vi "CW_change.vi"() -> ()   [LabVIEW 2020]
uses:
  SubVI/Fitting/fit.ctl
  SubVI/Microwave/mw.ctl
  SubVI/Fitting/fit_result.ctl
  <vilib>/Analysis/baseanly.llb/Mean (DBL).vi
  labview_control/Global  Parameter.vi
  labview_control/LaoJi/NI CTR/NI DAQ Counter.lvlib
  Labview Library/Libraries/ASG8100CY/ASG8100CY.lvlib
  <vilib>/Analysis/NI_AALBase.lvlib
panel:
  in  "milliseconds to wait":u32=20
  in  "等待时间（毫秒）":u32=200
  in  "Thre 2":dbl=82866.0 caption="counts" format="%0.2f"
  out "Fre step":ext
  out "Stop Ref":refnum<vi>
  out "x-y 2":dbl
  out "x-y":dbl
  out "error out":errorcluster
  in  "pulse loop times":i32=900000 format="%#.4p"
  out "Signal data":ext[](array[numeric])
  out "Pro data":ext[](array[numeric])
  out "Ref data":ext[](array[numeric])
  out "Fre sequence":ext[](array[numeric])=[1150.0, 1160.0, 1170.0, 1180.0, 1190.0, 1200.0, 1210.0, 1220.0, 1230.0, 1240.0, 1250.0, 1260.0, 1270.0, 1280.0, 1290.0, 1300.0, 1310.0, 1320.0, 1330.0, 1340.0, 1350.0, 1360.0, 1370.0, 1380.0, 1390.0, 1400.0, 1410.0, 1420.0, 1430.0, 1440.0, 1450.0, 1460.0, 1470.0, 1480.0, 1490.0, 1500.0, 1510.0, 1520.0, 1530.0, 1540.0, 1550.0, 1560.0, 1570.0, 1580.0, 1590.0, 1600.0, 1610.0, 1620.0, 1630.0, 1640.0]
  out "fit result":T1={"1/2pi"=0.0, "pi"=0.0, "3/2pi"=0.0, "T2"=0.0, "freq"=2869.360957411588, "gap"=0.0, "snr"=10.094902959180725, "width 2"=0.0, "freq 2"=0.0}
  out "element":dbl=2870.0
  in  "?":T2(tab)
  in  "CW Sequence Filepath":path=path "F:/Labview_Control_SIC/ASG8100_Labview/cw.pulse"
  in  "cw loop times":i32=1000 format="%#.4p"
  in  "Pulse Sequence Filepath":path
  out "freq":dbl
  out "freq 3":dbl=1434.680478705794
  out "Reference":cluster{"Fre sequence":ext[], "Ref data":ext[]}(graph)
  out "Signal":T3(graph) caption="signal"
  out "Sum of 3 Gaussians":T4(graph) caption="CW"
  out "Probability":cluster{"Fre sequence":ext[], "Pro data":ext[]}(graph) caption="CW"
  in  "?":T5=enum."cw_single_peak"
  in  "Limit":T6={"width threshold -"=2.0, "width threshold +"=8.0, "contrast threshold"=0.03, "fit error threshold"=3.0}
  out "NV or not?":bool
  in  "MW":T7={"mw_source"=enum."rigol", "MW Source IP Address"="192.168.3.3", "Remote Port"=5025, "Frequency(MHz)"=1500.0, "Power(dBm)"=-20.0}
  in  "setting section":T8={"mode"=enum."CW", "Start freq"=1150.0, "Stop freq"=1650.0, "Num Pts"=50, " dBm"=-15.0, "average"=3000, "Reference"=1}
  in  "Final Power dBm":dbl=-30.0
  out "fit frequency":dbl=2869.360957411588
  in  "freq offset":dbl
  in  "ratio":dbl=0.7
  out "Peak Count Rate":dbl=393329.896735343
  out "threshold":dbl=68289.2
  out "mean":dbl=82866.0 caption="counts" format="%0.2f"
  in  "autotrace\nbefore CW?":bool=TRUE
  in  "scan width":dbl=50.0
  in  "auto change":bool
  in  "drift(MHz)":ext
  in  "name":string="NV_1.17_"
  out "cw path":path=path "D:/cw data/NV_1.17_4_2_2021_5_06_50_PM.txt"
  in  "?":bool
  out "gap":dbl
  out "freq 2":dbl
  out "full name":string="NV_1.17_4_2_2021_5_06_50_PM"
  out "1-D Array of Real":dbl[](array[numeric])
  out "System Waveform Chart":u32[](graph)
  out "CW Chart":dbl(graph)
  out "Signal and Ref":cluster{"Numeric":dbl, "Numeric":dbl}(graph)
  # "auto change section"
  # "autotrace section"
  # "final section"
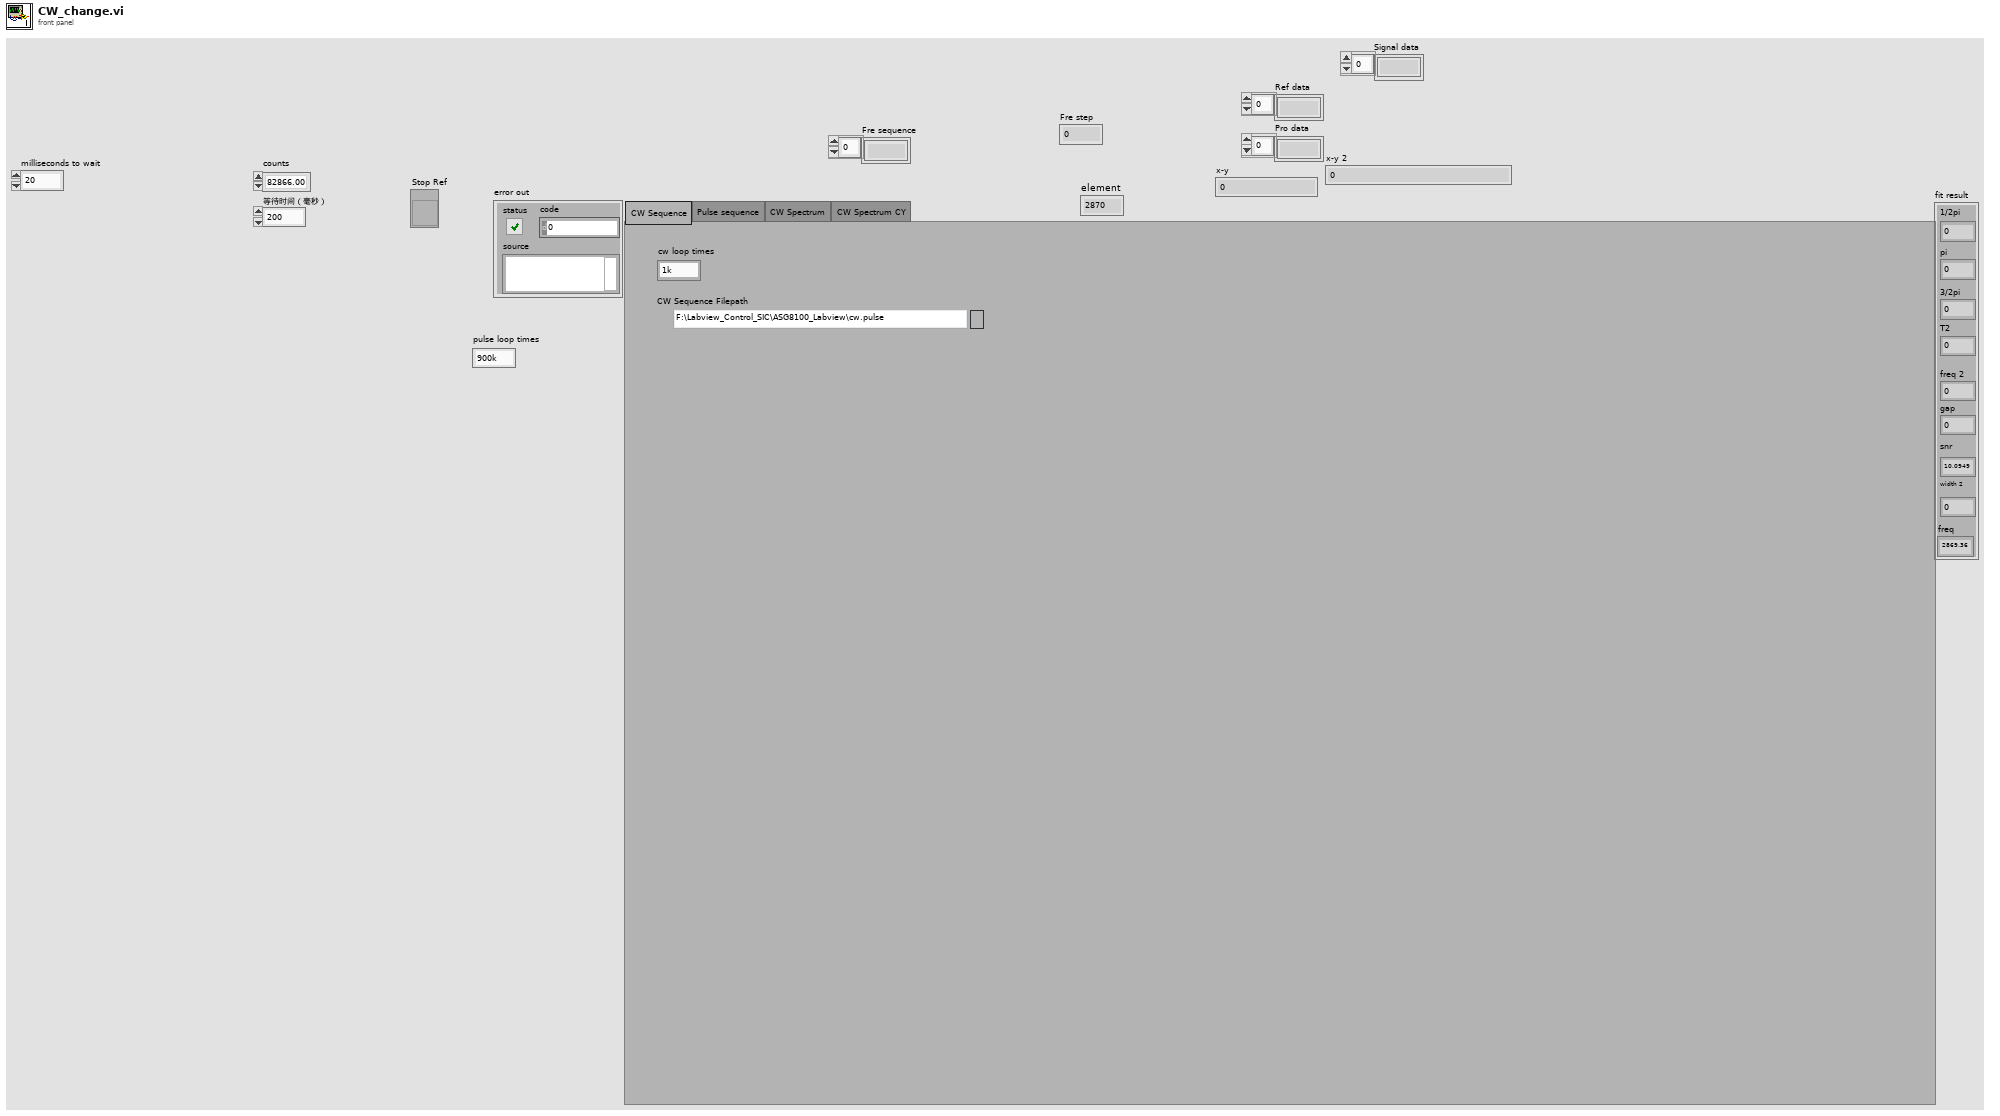
[diagram p1: front panel]
types:
  T1 = typedef "fit_result.ctl" = cluster{"1/2pi":dbl, "pi":dbl, "3/2pi":dbl, "T2":dbl, "freq":dbl, "gap":dbl, "snr":dbl, "width 2":dbl, "freq 2":dbl}
  T2 = enum32{"CW Sequence", "Pulse sequence", "CW Spectrum", "CW Spectrum CY"}
  T3 = cluster{"Fre sequence":ext[], "Signal data":ext[]}
  T4 = cluster{"Fre sequence":ext[], "best nonlinear fit":dbl[]}[]
  T5 = typedef "fit.ctl" = enum16{"autotrace", "T2", "sindamp", "cw_N14", "cw_single_peak", "cw_two_peak", "T2N"}
  T6 = cluster{"width threshold -":dbl, "width threshold +":dbl, "contrast threshold":dbl, "fit error threshold":dbl}
  T7 = typedef "mw.ctl" = cluster{"mw_source":enum16{"rigol", "stanford", "apsin", "hittle"}, "MW Source IP Address":string, "Remote Port":u16, "Frequency(MHz)":dbl, "Power(dBm)":dbl}
  T8 = cluster{"mode":enum16{"Pulsed", "CW"}, "Start freq":ext, "Stop freq":ext, "Num Pts":i32, " dBm":dbl, "average":i32, "Reference":i32}
  T9 = enum32{"Bad", "Idle", "Run top level", "Running"}
  T10 = cluster{"Fre sequence":ext[], "History Data":dbl[]}
  T11 = cluster{"1/2pi":dbl, "pi":dbl, "3/2pi":dbl, "T2":dbl, "freq":dbl, "p1":dbl, "p2":dbl, "error":dbl, "width 2":dbl}
  T12 = cluster{"Fre sequence":ext[], "best nonlinear fit":dbl[]}
  T13 = cluster{"Fre sequence":ext[], "History Data":dbl[]}[]
  T14 = typedef "imagedata.ctl" = cluster{"image type":i32, "image depth":i32, "image":u8[], "mask":u8[], "colors":u32[], "Rectangle":cluster{"left":i16, "top":i16, "right":i16, "bottom":i16}}
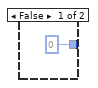
[diagram p2: hidden frame]
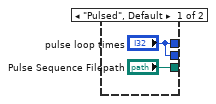
[diagram p5: hidden frame]
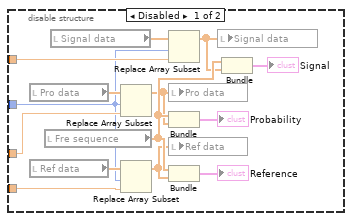
[diagram p6: hidden frame]
diagram:
  (unwired) dbl[] [] ("History Data")
  (unwired) dbl[] [] ("History Data")
  n1 = disable-structure shown="Disabled" {
    disable-tunnel: [w16 _] -> w12
    frame Disabled {
      n2 = flat-sequence {
        tunnel: [w17] -> w16
        frame #0 {
          n3 = local read "fit frequency"() -> (w18:dbl)
          n4 = Add(x=w18, y="drift(MHz)") -> (x+y=w20:ext)
          n5 = case shown="True" "auto change" {
            tunnel: w20 -> [_ w38]
            tunnel: [0 w23] -> w17
            frame False {
            }
            frame True {
              n6 = flat-sequence {
                tunnel: w38 -> [w46]
                tunnel: [w45] -> w37
                tunnel: [w44] -> w35
                tunnel: [w43] -> w33
                tunnel: [w42] -> w30
                tunnel: [w41] -> w29
                tunnel: [w40] -> w26
                tunnel: [w39] -> w25
                tunnel: w37 -> [w56]
                tunnel: [w56] -> w36
                tunnel: w35 -> [w55]
                tunnel: [w55] -> w34
                tunnel: w33 -> [w54]
                tunnel: [w54] -> w32
                tunnel: [w53] -> w31
                tunnel: w30 -> [w53]
                tunnel: w29 -> [w52]
                tunnel: [w52] -> w28
                tunnel: [w51] -> w27
                tunnel: w26 -> [w51]
                tunnel: w25 -> [w50]
                tunnel: [w50] -> w24
                tunnel: w36 -> [w58]
                tunnel: w34 -> [w59]
                tunnel: w32 -> [w65]
                tunnel: w31 -> [w64]
                tunnel: w28 -> [w63]
                tunnel: w27 -> [w62]
                tunnel: w24 -> [w61]
                tunnel: [0] -> w23
                frame #0 {
                  n7 = local read "setting section"() -> (w43:T8)
                  n8 = Divide(x="scan width", y=2) -> (x/y=w47:dbl)
                  n9 = Unbundle By Name(w43) -> ("mode"=w42:enum16{"Pulsed", "CW"}, "Num Pts"=w41:i32, "dBm"=w40:dbl, "average"=w39:i32)  [unwired: 2 out]
                  n10 = Subtract(x=w46, y=w47) -> (x-y=w44:ext)
                  n11 = Add(x=w46, y=w47) -> (x+y=w45:ext)
                }
                frame #1 {
                }
                frame #2 {
                  n12 = Bundle By Name(cluster=w65, "mode"=w64, "Num Pts"=w63, "Start freq"=w59, "Stop freq"=w58, "dBm"=w62, "average"=w61) -> (w60:T8)
                  n13 = local write "setting section"(w60) -> ()
                }
              }
            }
          }
        }
      }
    }
    frame Enabled {
    }
  }
  n14 = flat-sequence {
    tunnel: ["setting section"] -> w13
    tunnel: w12 -> [_]
    frame #0 {
    }
  }
  n15 = Unbundle By Name(w13) -> ("Num Pts"=w9:i32, "Start freq"=w4:ext, "Stop freq"=w5:ext)
  n16 = Increment(x=w9) -> (x+1=w8:i32)
  n17 = Subtract(x=w5, y=w4) -> (x-y=w15:ext)
  n18 = Divide(x=w15, y=w9) -> (x/y=w6:ext)
  "Fre step" <- w6
  n19 = flat-sequence {
    tunnel: [TRUE] -> w7
    frame #0 {
      n20 = control-ref of="?"() -> (→"Stop Ref":refnum<vi>)
    }
  }
  n21 = property on="CW Chart" class="WFChart (strict)"("XScale.Multiplier"=w6, "XScale.Maximum"=w5, "XScale.Minimum"=w4, "XScale.Offset"=w4, "History Data"=dbl[] []) -> ()  [unwired: 2 in, 2 out]
  n22 = property on="Signal and Ref" class="WFChart (strict)"("XScale.Multiplier"=w6, "XScale.Maximum"=w5, "XScale.Minimum"=w4, "History Data"=cluster{"Numeric":dbl, "Numeric":dbl}[] [], "XScale.Offset"=w4) -> ()  [unwired: 2 in, 2 out]
  n23 = for {
    N: w8 -> [_]
    tunnel: w4 -> [w72]
    tunnel: w6 -> [w73]
    tunnel: [w69] -> w11 mode=indexing
    i -> [w70]
    n24 = Multiply(x=w70, y=w73) -> (x*y=w71:ext)
    n25 = Add(x=w72, y=w71) -> (x+y=w69:ext)
  }
  "Fre sequence" <- w11
  n26 = Multiply(x=0.0 ("元素"), y=w11) -> (x*y=w10:ext[])
  n27 = flat-sequence {
    tunnel: w10 -> [w75]
    tunnel: w7 -> [_]
    tunnel: [w210] -> w2
    tunnel: w2 -> [w218]
    frame #0 {
      n28 = flat-sequence {
        frame #0 {
          n29 = case shown="True" "autotrace\nbefore CW?" {
            frame False {
            }
            frame True {
              n30 = local read "CW Sequence Filepath"() -> (w80:path)
              n31 = call "ThreeAxis AutoTrace.vi"() -> ("error out"=w81:errorcluster, "Peak Count"=w82:dbl[])  [unwired: 8 in, 2 out]
              n32 = call "Load By File.vi"("error in"=w81, "File Path"=w80) -> ("error out"=w79:errorcluster)  [unwired: 8 in, 1 out]
              n33 = Index Array(array=w82, index=2) -> (element=w83:dbl)
              n34 = call "ASG start playing.vi"("error in"=w79, "Loop Time"=0) -> ("error out"=w84:errorcluster)  [unwired: 8 in, 1 out]
              n35 = while {
                shift-right: [w95] -> w86
                shift-left: w83 -> [w92]
                tunnel: w84 -> [w90]
                shift-right: [w89] -> _
                shift-left: _ -> [_]
                stop <- w91 stop-if-true
                (unwired) 2 ("index")
                n36 = flat-sequence {
                  tunnel: w90 -> [w98]
                  tunnel: [w98] -> w88
                  tunnel: [w101] -> w96
                  tunnel: [w99] -> w89
                  tunnel: w88 -> [w100]
                  frame #0 {
                    n37 = Wait (ms)(milliseconds to wait="milliseconds to wait") -> ()  [unwired: 1 out]
                  }
                  frame #1 {
                    n38 = call "ThreeAxis AutoTrace.vi"("error in"=w100) -> ("error out"=w99:errorcluster, "Peak Count"=w101:dbl[])  [unwired: 7 in, 2 out]
                  }
                }
                n39 = Index Array(array=w96) -> (element=w95:dbl)  [unwired: 1 in]
                n40 = Multiply(x=w95, y=0.95) -> (x*y=w93:dbl)
                n41 = Greater?(x=w93, y=w92) -> (0:w91:bool)
              }
              "Peak Count Rate" <- w86
              n42 = Multiply(x="ratio", y=w86) -> (x*y=→"threshold":dbl)
            }
          }
        }
      }
      n43 = property on="System Waveform Chart" class="WFChart (strict)"("History Data"=u32[] []) -> ()  [unwired: 2 in, 2 out]
      "Ref data" <- w75
      "Pro data" <- w75
      "Signal data" <- w75
    }
    frame #1 {
      n44 = local read "setting section"() -> (w105:T8)
      n45 = Unbundle By Name(w105) -> ("mode"=w104:enum16{"Pulsed", "CW"})
      n46 = case shown="\"CW\"" w104 {
        tunnel: ["pulse loop times" "cw loop times"] -> w102
        tunnel: ["pulse loop times" "cw loop times"] -> _
        tunnel: ["Pulse Sequence Filepath" "CW Sequence Filepath"] -> w106
        frame "Pulsed", Default {
        }
        frame "CW" {
        }
      }
      n47 = local read "Fre sequence"() -> (w107:ext[])
      n48 = call "Load By File.vi"("File Path"=w106) -> ("error out"=w103:errorcluster)  [unwired: 9 in, 1 out]
      n49 = for {
        tunnel: w107 -> [w122] mode=indexing
        tunnel: w103 -> [w117]
        tunnel: w102 -> [w116]
        i -> [w118]
        stop <- "?" stop-if-true
        n50 = flat-sequence {
          tunnel: w122 -> [w128]
          tunnel: [w125] -> w114
          tunnel: [w146] -> w120
          tunnel: w117 -> [w139]
          tunnel: w116 -> [w136]
          tunnel: w114 -> [w134]
          tunnel: [w147] -> w123
          tunnel: w120 -> [w147]
          tunnel: w118 -> [w157]
          tunnel: w123 -> [w155]
          tunnel: [w151] -> w115
          tunnel: [w148] -> w113
          tunnel: w115 -> [w183]
          tunnel: w113 -> [w179]
          tunnel: [w178] -> w112
          tunnel: w112 -> [w186]
          frame #0 {
            n51 = local read "setting section"() -> (w124:T8)
            n52 = Unbundle By Name("MW") -> ("mw_source"=w131:enum16{"rigol", "stanford", "apsin", "hittle"}, "MW Source IP Address"=w130:string, "Remote Port"=w129:u16)
            n53 = Unbundle By Name(w124) -> ("dBm"=w127:dbl)
            n54 = Bundle By Name(cluster="MW", "mw_source"=w131, "MW Source IP Address"=w130, "Remote Port"=w129, "Frequency(MHz)"=w128, "Power(dBm)"=w127) -> (w126:T7)
            n55 = call <vilib>:"High Resolution Relative Seconds.vi"() -> ("relative seconds"=w125:dbl)
            n56 = call "MW setup.vi"("mw"=w126) -> ()  [unwired: 9 in, 2 out]
          }
          frame #1 {
            n57 = call <vilib>:"High Resolution Relative Seconds.vi"() -> ("relative seconds"=w135:dbl)
            n58 = Subtract(x=w135, y=w134) -> (x-y=→"x-y 2":dbl)
            n59 = Multiply(x=w136, y=4) -> (x*y=w137:i32)
            n60 = call "Init Finite Sampling.vi"("error in (no error)"=w139, "Num of Sample"=w137) -> ("error out"=w140:errorcluster)  [unwired: 9 in]
            n61 = call "ASG start playing.vi"("error in"=w140, "Loop Time"=w136) -> ("error out"=w141:errorcluster)  [unwired: 8 in, 1 out]
            n62 = call "Read Finite Sampling.vi"("error in (no error)"=w141, "Samples to Read"=w137) -> ("error out"=w143:errorcluster, "Sample Array"=w146:u32[])  [unwired: 7 in, 1 out]
            "System Waveform Chart" <- w146
            n63 = call "Stop Finite Sampling.vi"("error in (no error)"=w143) -> ("error out"=w144:errorcluster)  [unwired: 10 in]
            n64 = call "ASG stop playing.vi"("error in"=w144) -> ("error out"=w142:errorcluster)  [unwired: 9 in, 1 out]
            n65 = Merge Errors(w142) -> (→"error out":errorcluster)
          }
          frame #2 {
          }
          frame #3 {
            n66 = To Double Precision Float(number=w155) -> (double precision float=w154:dbl[])
            n67 = Decimate 1D Array(w154) -> (w152:dbl[], w149:dbl[])
            n68 = Add Array Elements(numeric array=w152) -> (sum=w158:dbl)
            n69 = Subtract(x=w152, y=w149) -> (x-y=w156:dbl[])
            n70 = call-poly <vilib>:"Mean.vi"("X"=w149) -> ("mean"=w148:dbl)  [unwired: 1 out]
            n71 = Add Array Elements(numeric array=w156) -> (sum=w153:dbl)
            n72 = Add Array Elements(numeric array=w149) -> (sum=w150:dbl)
            n73 = Divide(x=w153, y=w150) -> (x/y=w159:dbl)
            n74 = disable-structure shown="Enabled" {
              disable-tunnel: w159 -> [w172 w174]
              disable-tunnel: w158 -> [w169 w177]
              disable-tunnel: w157 -> [w168 _]
              disable-tunnel: w150 -> [w167 w176]
              frame Disabled {
                n75 = local read "Pro data"() -> (w173:ext[])
                n76 = local read "Ref data"() -> (w171:ext[])
                n77 = local read "Fre sequence"() -> (w166:ext[])
                n78 = local read "Signal data"() -> (w170:ext[])
                n79 = Replace Array Subset(array=w173, new element=w172, index=w168) -> (w164:ext[])
                n80 = Replace Array Subset(array=w171, new element=w167, index=w168) -> (w165:ext[])
                n81 = Replace Array Subset(array=w170, new element=w169, index=w168) -> (w163:ext[])
                n82 = local write "Pro data"(w164) -> ()
                n83 = Bundle("Fre sequence"=w166, "Pro data"=w164) -> (→"Probability":cluster{"Fre sequence":ext[], "Pro data":ext[]})  [unwired: 1 in]
                n84 = local write "Ref data"(w165) -> ()
                n85 = Bundle("Fre sequence"=w166, "Ref data"=w165) -> (→"Reference":cluster{"Fre sequence":ext[], "Ref data":ext[]})  [unwired: 1 in]
                n86 = local write "Signal data"(w163) -> ()
                n87 = Bundle("Fre sequence"=w166, "Signal data"=w163) -> (→"Signal":T3)  [unwired: 1 in]
              }
              frame Enabled {
                n88 = Bundle("Numeric"=w177, "Numeric"=w176) -> (→"Signal and Ref":cluster{"Numeric":dbl, "Numeric":dbl})  [unwired: 1 in]
                "CW Chart" <- w174
              }
            }
            n89 = call <vilib>:"High Resolution Relative Seconds.vi"() -> ("relative seconds"=w151:dbl)
          }
          frame #4 {
            n90 = call <vilib>:"High Resolution Relative Seconds.vi"() -> ("relative seconds"=w184:dbl)
            n91 = local read "threshold"() -> (w181:dbl)
            n92 = Subtract(x=w184, y=w183) -> (x-y=→"x-y":dbl)
            n93 = Less?(x=w179, y=w181) -> (x < y?=w185:bool)
            n94 = Less?(x=w179, y="Thre 2") -> (x < y?=w178:bool)
            n95 = case shown="True" w185 {
              frame False {
              }
              frame True {
                n96 = call "ThreeAxis AutoTrace.vi"() -> ()  [unwired: 8 in, 4 out]
              }
            }
            "mean" <- w179
          }
          frame #5 {
            n97 = case shown="True" w186 {
              frame False {
              }
              frame True {
                n98 = local read "CW Sequence Filepath"() -> (w191:path)
                n99 = call "Load By File.vi"("File Path"=w191) -> ("error out"=w190:errorcluster)  [unwired: 9 in, 1 out]
                n100 = call "ASG start playing.vi"("error in"=w190, "Loop Time"=0) -> ("error out"=w187:errorcluster)  [unwired: 8 in, 1 out]
                n101 = call "ThreeAxis AutoTrace.vi"("error in"=w187) -> ("error out"=w188:errorcluster)  [unwired: 7 in, 3 out]
                n102 = call "ASG stop playing.vi"("error in"=w188) -> ()  [unwired: 9 in, 2 out]
              }
            }
          }
          frame #6 {
            n103 = disable-structure shown="Enabled" {
              frame Enabled {
                n104 = Wait (ms)(milliseconds to wait="等待时间（毫秒）") -> ()  [unwired: 1 out]
              }
              frame Disabled {
              }
            }
          }
        }
        n105 = Wait (ms)(milliseconds to wait=u32 10 ("等待时间（毫秒）")) -> ()  [unwired: 1 out]
      }
    }
    frame #2 {
      n106 = local read "Fre sequence"() -> (w195:ext[])
      n107 = property on="CW Chart" class="WFChart (strict)"() -> ("History Data"=w193:dbl[])  [unwired: 2 in, 2 out]
      n108 = Array Max & Min(array=w193) -> (min index (indices)=w197:i32)  [unwired: 3 out]
      n109 = Bundle("Fre sequence"=w195, "History Data"=w193) -> (w216:T10)  [unwired: 1 in]
      n110 = call "Fitpulse.vi"("fit function"="?", "X"=w195, "Y"=w193) -> ("best nonlinear fit"=w206:dbl[], "export parameter"=w208:T11, "fit result"=w205:T1)  [unwired: 4 in, 2 out]
      "fit result" <- w205
      n111 = Unbundle By Name(w205) -> ("gap"=→"gap":dbl, "freq 2"=w202:dbl, "freq"=w201:dbl)
      "freq 2" <- w202
      n112 = Unbundle By Name(w208) -> ("freq"=w194:dbl)
      "fit frequency" <- w194
      "freq" <- w194
      n113 = Index Array(array=w195, index=w197) -> (element=→"element":ext)
      n114 = Array Max & Min(array=w206) -> (min value=w213:dbl)  [unwired: 3 out]
      n115 = Bundle("Fre sequence"=w195, "best nonlinear fit"=w206) -> (w215:T12)  [unwired: 1 in]
      n116 = Unbundle By Name("Limit") -> ("contrast threshold"=w211:dbl)
      n117 = Add(x=w194, y="freq offset") -> (x+y=w210:dbl)
      n118 = Add(x=w202, y=w201) -> (x+y=w200:dbl)
      n119 = Build Array(w215, w216) -> (→"Sum of 3 Gaussians":T13)
      n120 = Absolute Value(x=w213) -> (abs(x)=w212:dbl)
      n121 = Greater Or Equal?(x=w212, y=w211) -> (x >= y?=→"NV or not?":bool)
      n122 = Divide(x=w200, y=2.0) -> (x/y=→"freq 3":dbl)
    }
    frame #3 {
      n123 = local read "MW"() -> (w220:T7)
      n124 = Unbundle By Name(w220) -> ("mw_source"=w221:enum16{"rigol", "stanford", "apsin", "hittle"}, "MW Source IP Address"=w222:string, "Remote Port"=w223:u16)  [unwired: 2 out]
      n125 = Bundle By Name(cluster=w220, "mw_source"=w221, "MW Source IP Address"=w222, "Remote Port"=w223, "Frequency(MHz)"=w218, "Power(dBm)"="Final Power dBm") -> (w224:T7)
      n126 = call "MW setup.vi"("mw"=w224) -> ()  [unwired: 9 in, 2 out]
    }
    frame #4 {
      n127 = local read "Fre sequence"() -> (w233:ext[])
      n128 = local read "Pro data"() -> (w234:ext[])
      n129 = global read "Global  Parameter.vi" "NV name"() -> (w227:string)
      n130 = script code="x=x';\ny=y';\nft = fittype('A1*exp(-((x-freq1)/sigma1)^2)+A2*exp(-((x-freq2)/sigma2)^2)+y0','independent','x', 'dependent','y');\n[A1_ini,A2_ini,freq1_ini,freq2_ini]=ini_2_peak(x,y);\n    sigma_ini = 0.5;%MHz\n    y0_ini = max(y);\n    opts = fitoptions('Method', 'NonlinearLeastSquares');\n    opts.StartPoint = [A1_ini A2_ini freq1_ini freq2_ini sigma_ini sigma_ini y0_ini];\n    f = fit(x,y,ft,opts);\n    err = confint(f);  \n    \n    if f.freq1<f.freq2\n      freqs(1) = f.freq1;\n      freqs(2) = err(2,3)-err(1,3);   \n      freqs(3) = f.freq2;\n      freqs(4) = err(2,4)-err(1,4);\n    else\n      freqs(3) = f.freq1;\n      freqs(4) = err(2,3)-err(1,3);   \n      freqs(1) = f.freq2;\n      freqs(2) = err(2,4)-err(1,4);  \n    end"("x"=w233, "y"=w234) -> ("??"=w226:errorcluster, "freqs"=w228:dbl[])  [unwired: 1 in]
      "1-D Array of Real" <- w228
      n131 = global read "Global  Parameter.vi" "fit frequency list"() -> (w230:dbl[][])
      n132 = call <vilib>:"Clear Errors.vi"("error in (no error)"=w226) -> ()  [unwired: 5 in, 2 out]
      n133 = Scan From String(format string="NV_%d", input string=w227) -> (output 1=w229:i32)  [unwired: 3 in, 3 out]
      n134 = Insert Into Array(array=w228, new element=w229) -> (w231:dbl[])  [unwired: 1 in]
      n135 = Insert Into Array(array=w230, new element=w231) -> (w232:dbl[][])  [unwired: 2 in]
      n136 = global write "Global  Parameter.vi" "fit frequency list"(w232) -> ()
    }
    frame #5 {
      n137 = flat-sequence {
        tunnel: [w237] -> w235
        tunnel: w235 -> [w248]
        frame #0 {
          n138 = global read "Global  Parameter.vi" "NV name"() -> (w236:string)
          n139 = local write "name"(w236) -> ()
        }
        frame #1 {
          n140 = case shown="\"Run top level\", Default" T9."Run top level" ("Exec.State") {
            frame "Run top level", Default {
              n141 = global read "Global  Parameter.vi" "cw path"() -> (w243:path)
              n142 = local write "cw path"(w243) -> ()
            }
            frame "Idle" {
            }
          }
          n143 = Format Date/Time String(time format string (%c)="%Y_%m_%H_%M_%S") -> (date/time string=w240:string)  [unwired: 2 in]
          n144 = Concatenate Strings(w240, "_" ("string"), "name") -> (w237:string)
          "full name" <- w237
        }
        frame #2 {
          n145 = invoke class="TabCtl (strict)" method="Get Image"() -> ("image data"=w249:T14)  [unwired: 6 in, 5 out]
          n146 = global read "Global  Parameter.vi" "cw path"() -> (w247:path)
          n147 = local read "Fre sequence"() -> (w245:ext[])
          n148 = local read "Pro data"() -> (w244:ext[])
          n149 = call "savepic.vi"("image data"=w249, "name"=w248, "Path"=w247) -> ()  [unwired: 7 in, 2 out]
          n150 = Build Array(w245, w244) -> (w251:ext[][])
          n151 = Transpose 2D Array(2D array=w251) -> (transposed array=w250:ext[][])
          n152 = call "savetxt.vi"("2D data"=w250, "name"=w248, "path"=w247) -> ("saved path"=→"cw path":path)  [unwired: 8 in]
        }
        frame #3 {
          n153 = Get Date/Time In Seconds() -> (seconds since 1Jan1904=w252:timestamp)
          n154 = global write "Global  Parameter.vi" "auto cw time"(w252) -> ()
        }
      }
    }
  }
